vi "golpi_mpc_command.vi"(5 "clear function cache before command? (False)":bool, 7 "timeout [ms]":u32=10000, 8 "error in":errorcluster, 10 "command":string, 11 "GOLPI ref in":T1={"pipe handle"={"lv_proc.dll file path"=path "", "process instance handle"=[], "debug mode"=FALSE, "debug data"=[]}, "fast read timeout [ms]"=500, "fast read settle time [ms]"=10, "fast read to multiple [ms]"=1, "max elements per input line"=100, "slow read timeout [ms]"=5000, "stdin double format specifier"="%_16e", "max elements per stdout output column"=100, "console mode bitstream"=FALSE, "bitstream first read timeout [ms]"=1000, "bitstream read timeout [ms]"=50, "struct transfer possible"=FALSE, "matlab mode"=FALSE}) -> (0 "error out":errorcluster, 2 "read buffer":string, 3 "GOLPI ref. out":T1={"pipe handle"={"lv_proc.dll file path"=path "", "process instance handle"=[], "debug mode"=FALSE, "debug data"=[]}, "fast read timeout [ms]"=500, "fast read settle time [ms]"=10, "fast read to multiple [ms]"=1, "max elements per input line"=100, "slow read timeout [ms]"=5000, "stdin double format specifier"="%_16e", "max elements per stdout output column"=100, "console mode bitstream"=FALSE, "bitstream first read timeout [ms]"=1000, "bitstream read timeout [ms]"=50, "struct transfer possible"=FALSE, "matlab mode"=FALSE})   [LabVIEW 2018, in "GOLPI Multi Process.lvlib"]
doc: "Multi-process GOLPI command. Call this when you need to execute GOLPI command (equivalent of GOLPI write) but it will also wait for command execution for a given timeout. Then it will return command text output.\nOptionally it will prepend function cache clear command. This is useful for debug because sometimes Octave does not update called functions even if they changed on the disk."
uses:
  GOLPI Multi Process.lvlib
  GOLPI Library.lvlibp/Public/GOLPI reference Type Def.ctl
  GOLPI Library.lvlibp/LV Process source distribution/Pipe Handle.ctl
  GOLPI Library.lvlibp
  GOLPI Library.lvlibp/LV Process source distribution/LV Process library.lvlib
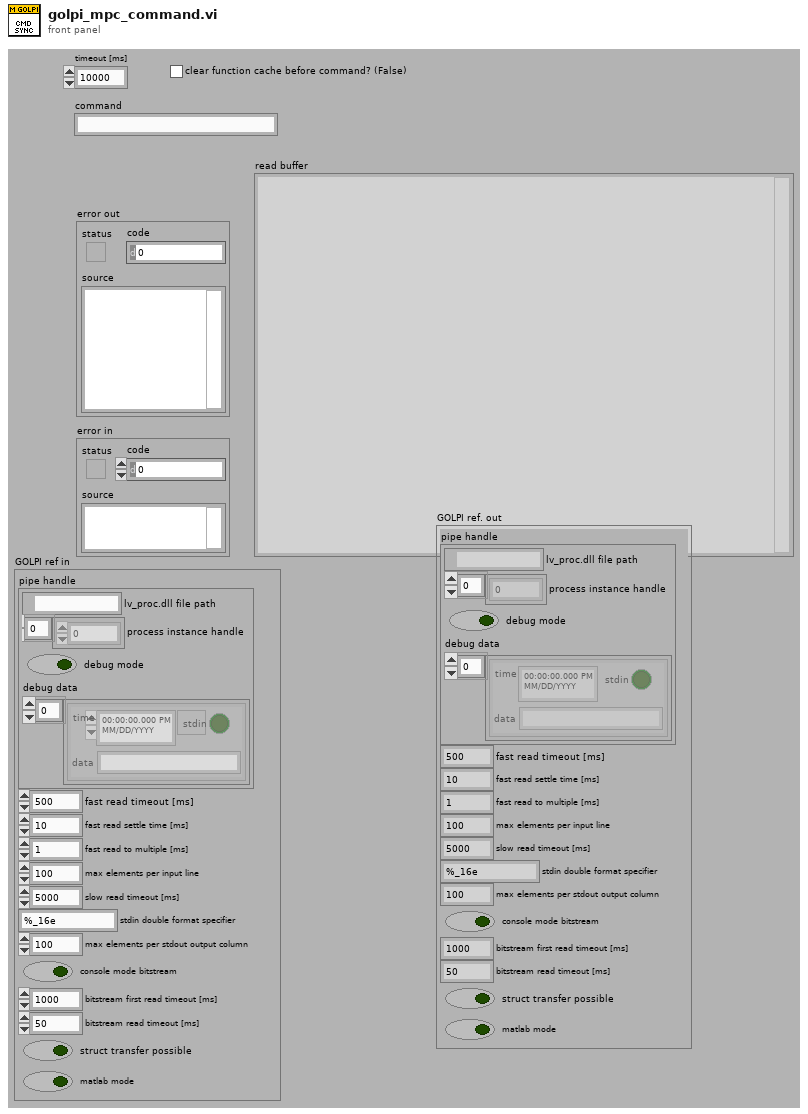
[diagram p1: front panel]
types:
  T1 = typedef "GOLPI Library.lvlibp/GOLPI reference Type Def.ctl" = cluster{"pipe handle":T2, "fast read timeout [ms]":u32, "fast read settle time [ms]":u32, "fast read to multiple [ms]":u32, "max elements per input line":u32, "slow read timeout [ms]":u32, "stdin double format specifier":string, "max elements per stdout output column":u32, "console mode bitstream":bool, "bitstream first read timeout [ms]":u32, "bitstream read timeout [ms]":u32, "struct transfer possible":bool, "matlab mode":bool}
  T2 = typedef "GOLPI Library.lvlibp/LV Process library.lvlib/Pipe Handle.ctl" = cluster{"lv_proc.dll file path":path, "process instance handle":u32[], "debug mode":bool, "debug data":cluster{"time":timestamp, "stdin":bool, "data":string}[]}
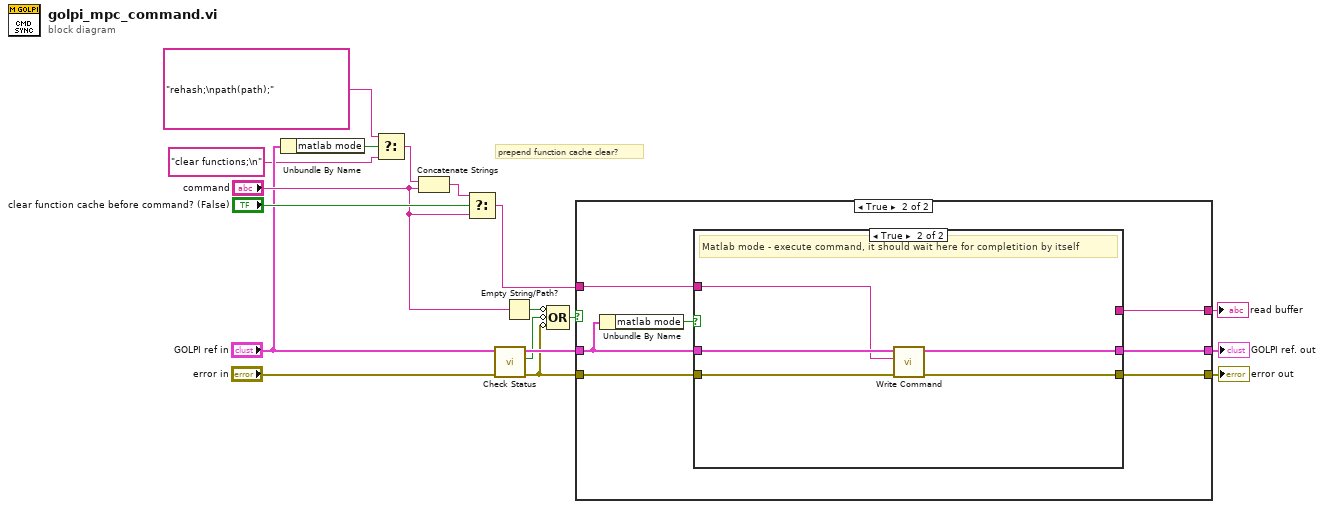
[diagram p0: block diagram]
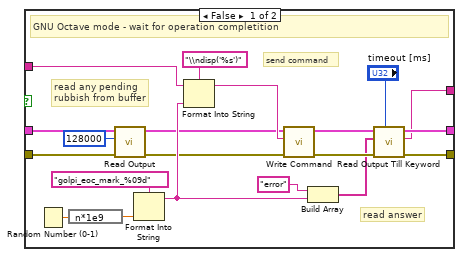
[diagram p3: hidden frame]
diagram:
  # "prepend function cache clear?"
  n1 = Unbundle By Name("GOLPI ref in") -> ("matlab mode"=w4:bool)
  n2 = Select(t="rehash;\npath(path);" ("string"), s=w4, f="clear functions;\n" ("string")) -> (s? t:f=w3:string)
  n3 = Concatenate Strings(w3, "command") -> (w8:string)
  n4 = Select(t=w8, s="clear function cache before command? (False)", f="command") -> (s? t:f=w9:string)
  n5 = call "Check Status.vi"("error in"="error in", "GOLPI ref. in"="GOLPI ref in") -> ("error out"=w11:errorcluster, "exited?"=w12:bool, "GOLPI ref. out"=w15:T1)  [unwired: 7 in]
  n6 = Empty String/Path?(string/path="command") -> (empty?=w13:bool)
  n7 = Compound Arithmetic op=OR(invert w13, invert w12, invert w11) -> (w14:bool)
  n8 = case shown="True" w14 {
    tunnel: w11 -> [w20 w24]
    tunnel: w15 -> [w19 w22]
    tunnel: [w20 w27] -> w18
    tunnel: [w19 w26] -> w17
    tunnel: w9 -> [_ w25]
    tunnel: [_ w23] -> w6
    frame False {
    }
    frame True {
      n9 = Unbundle By Name(w22) -> ("matlab mode"=w21:bool)
      n10 = case shown="True" w21 {
        tunnel: [w44 w51] -> w27
        tunnel: [w43 w50] -> w26
        tunnel: w25 -> [w37 w48]
        tunnel: w24 -> [w33 w52]
        tunnel: [w29 _] -> w23
        tunnel: w22 -> [w28 w49]
        frame False {
          # "read answer"
          # "send command"
          # "read any pending\nrubbish from buffer"
          # "GNU Octave mode - wait for operation completition"
          n11 = Random Number (0-1)() -> (number: 0 to 1=w41:dbl)
          n12 = expression code="n*1e9"(w41) -> (w40:dbl)
          n13 = call "Read Output.vi"("error in"=w33, "byte count"=128000, "GOLPI ref. in"=w28) -> ("error out"=w31:errorcluster, "GOLPI ref. out"=w32:T1)  [unwired: 5 in, 2 out]
          n14 = Format Into String(format string="golpi_eoc_mark_%09d", w40) -> (resulting string=w35:string)  [unwired: 2 in, 1 out]
          n15 = Format Into String(format string="\\ndisp('%s')", initial string=w37, w35) -> (resulting string=w34:string)  [unwired: 1 in, 1 out]
          n16 = call "Write Command.vi"("error in"=w31, "command"=w34, "GOLPI ref. in"=w32) -> ("error out"=w47:errorcluster, "GOLPI ref. out"=w46:T1)  [unwired: 7 in]
          n17 = Build Array("error" ("keyword"), w35) -> (w39:string[])
          n18 = call "Read Output Till Keyword.vi"("timeout [ms]"="timeout [ms]", "error in"=w47, "keywords"=w39, "GOLPI ref. in"=w46) -> ("error out"=w44:errorcluster, "read buffer"=w29:string, "GOLPI ref. out"=w43:T1)  [unwired: 4 in, 1 out]
        }
        frame True {
          # "Matlab mode - execute command, it should wait here for completition by itself"
          n19 = call "Write Command.vi"("error in"=w52, "command"=w48, "GOLPI ref. in"=w49) -> ("error out"=w51:errorcluster, "GOLPI ref. out"=w50:T1)  [unwired: 7 in]
        }
      }
    }
  }
  "error out" <- w18
  "GOLPI ref. out" <- w17
  "read buffer" <- w6
